vi "pack.vi"(8 "error in (no error)":errorcluster, 11 "Wrapper in":refnum<class "Wrapper.lvclass">) -> (0 "error out":errorcluster, 2 "Packing":string, 3 "Wrapper out":refnum<class "Wrapper.lvclass">)   [LabVIEW 2018, in "Wrapper.lvclass"]
uses:
  Wrapper.lvclass
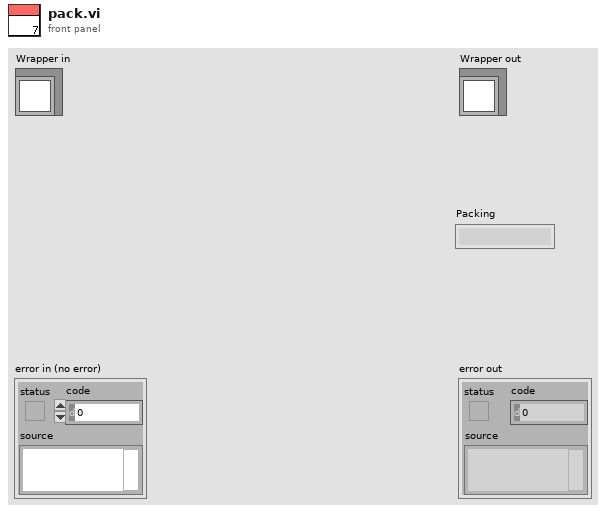
[diagram p1: front panel]
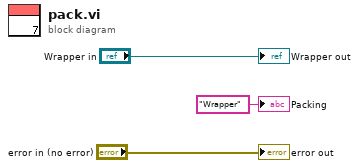
[diagram p0: block diagram]
diagram:
  "error out" <- "error in (no error)"
  "Wrapper out" <- "Wrapper in"
  "Packing" <- "Wrapper" ("Packing")
